vi "例4-18.vi"() -> ()   [LabVIEW 2019]
panel:
  out "LED灯":cluster{"红灯":bool, "绿灯":bool, "蓝灯":bool}
  in  "停止":bool
  in  "亮灯控制":enum16{"红色", "绿色", "蓝色"}(ring)
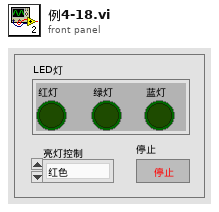
[diagram p1: front panel]
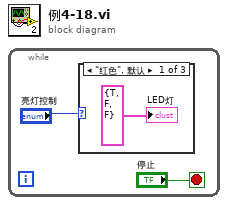
[diagram p0: block diagram]
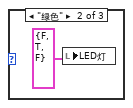
[diagram p2: hidden frame]
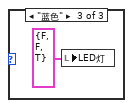
[diagram p3: hidden frame]
diagram:
  n1 = while {
    stop <- "停止" stop-if-true
    n2 = case shown="\"红色\", 默认" "亮灯控制" {
      frame "红色", Default {
        "LED灯" <- cluster{bool, bool, bool} {TRUE, FALSE, FALSE}
      }
      frame "绿色" {
        n3 = local write "LED灯"(cluster{bool, bool, bool} {FALSE, TRUE, FALSE}) -> ()
      }
      frame "蓝色" {
        n4 = local write "LED灯"(cluster{bool, bool, bool} {FALSE, FALSE, TRUE}) -> ()
      }
    }
  }
